vi "简易计算器的制作(上).vi"() -> ()   [LabVIEW 2018]
panel:
  out "连接的字符串":string
  in  "?":bool
  in  "?":bool
  in  "?":bool
  in  "?":bool
  in  "?":bool
  in  "?":bool
  in  "?":bool
  in  "?":bool
  in  "?":bool
  in  "?":bool
  in  "?":bool
  in  "?":bool
  in  "?":bool
  in  "?":bool
  in  "?":bool
  in  "?":bool
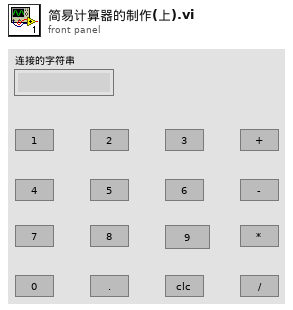
[diagram p1: front panel]
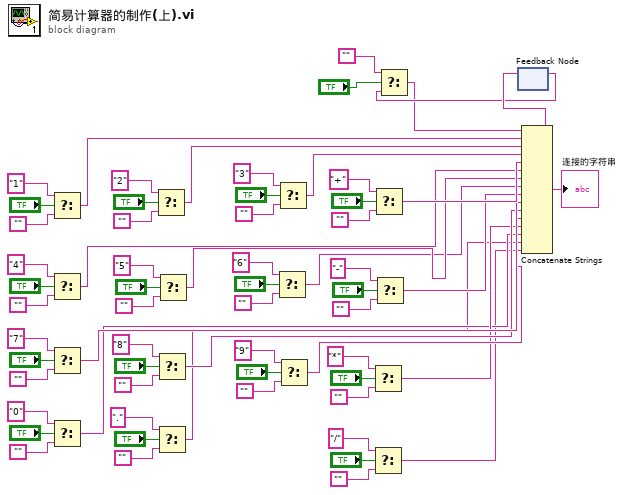
[diagram p0: block diagram]
diagram:
  n1 = Select(t="1", s="?", f="") -> (s? t:f=w19:string)
  n2 = Select(t="4", s="?", f="") -> (s? t:f=w15:string)
  n3 = Select(t="7", s="?", f="") -> (s? t:f=w11:string)
  n4 = Select(t="0", s="?", f="") -> (s? t:f=w7:string)
  n5 = Select(t="2", s="?", f="") -> (s? t:f=w18:string)
  n6 = Select(t="8", s="?", f="") -> (s? t:f=w10:string)
  n7 = Select(t=".", s="?", f="") -> (s? t:f=w6:string)
  n8 = Select(t="5", s="?", f="") -> (s? t:f=w14:string)
  n9 = Select(t="6", s="?", f="") -> (s? t:f=w13:string)
  n10 = Select(t="3", s="?", f="") -> (s? t:f=w17:string)
  n11 = Select(t="9", s="?", f="") -> (s? t:f=w9:string)
  n12 = Select(t="*", s="?", f="") -> (s? t:f=w8:string)
  n13 = Select(t="/", s="?", f="") -> (s? t:f=w5:string)
  n14 = Select(t="+", s="?", f="") -> (s? t:f=w16:string)
  n15 = Select(t="-", s="?", f="") -> (s? t:f=w12:string)
  n16 = feedback #1() -> (w2:string)  [unwired: 1 in]
  n17 = Select(t="", s="?", f=w2) -> (s? t:f=w1:string)
  n18 = Concatenate Strings(w1, w19, w18, w17, w16, w15, w14, w13, w12, w11, w10, w9, w8, w7, w6, w5) -> (w20:string)
  "连接的字符串" <- w20
  n19 = feedback-in #1(w20) -> ()
